vi "LNLS Control PS Data to LOCON_BIPOLAR_16BITS Data.vi"(8 "error in (no error)":errorcluster, 10 "PS Status":bool[](array[boolean]), 11 "PS Readings/Setpoints":dbl[](array[numeric])) -> (0 "error out":errorcluster, 3 "PS Readings/Setpoints LOCON Data":T1[](array[typedef]) {"status" format="%08b"})   [LabVIEW 2011, in "LNLS Control VIs.lvlib"]
uses:
  LNLS Control VIs.lvlib
  Types Definitions/Type LOCON_BIPOLAR_16BITS.ctl
  Type Definitions.lvlib
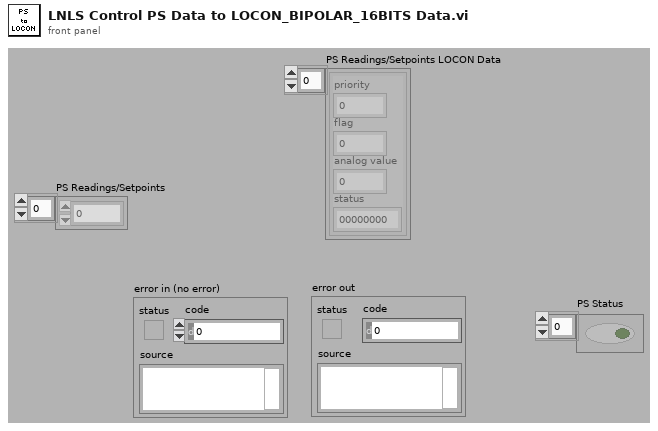
[diagram p1: front panel]
types:
  T1 = typedef "Type Definitions.lvlib/Type LOCON_BIPOLAR_16BITS.ctl" = cluster{"priority":u8, "flag":u8, "analog value":u16, "status":u8}
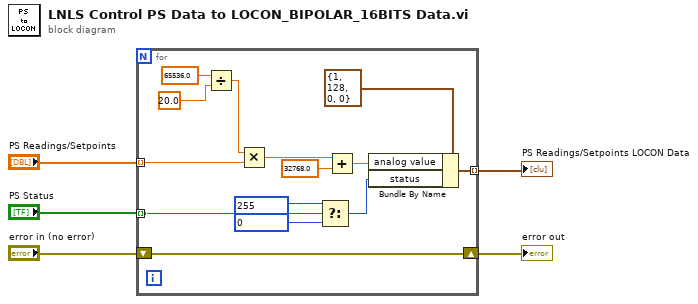
[diagram p0: block diagram]
diagram:
  n1 = for {
    tunnel: [w19] -> w2 mode=indexing
    shift-right: [w10] -> w4
    shift-left: "error in (no error)" -> [w10]
    tunnel: "PS Readings/Setpoints" -> [w7] mode=indexing
    tunnel: "PS Status" -> [w6] mode=indexing
    n2 = Divide(x=65536.0, y=20.0) -> (x/y=w9:dbl)
    n3 = Multiply(x=w9, y=w7) -> (x*y=w13:dbl)
    n4 = Select(t=u8 255, s=w6, f=u8 0 ("t")) -> (s? t:f=w18:u8)
    n5 = Add(x=w13, y=32768.0) -> (x+y=w11:dbl)
    n6 = Bundle By Name(cluster=T1 {"priority"=1, "flag"=128, "analog value"=0, "status"=0}, "analog value"=w11, "status"=w18) -> (w19:T1)
  }
  "PS Readings/Setpoints LOCON Data" <- w2
  "error out" <- w4
